vi "Actor.vi"(6 "Self Alias":string, 8 "Actor":refnum<class "Actor.lvclass">, 9 "Creator Attributes":T1, 10 "Queue of Created Init":refnum<queue>) -> ()   [LabVIEW 2020, in "jettl.lvlib" / "Actor.lvlib" / "Base Actor.lvclass"]
uses:
  Base Actor.lvclass
  Actor/Actor.lvclass
  Msg/Msg.lvclass
  Last Ack Msg/Last Ack Msg.lvlib
  Implemented Msgs.ctl
  Actor.lvlib
  Attributes.ctl
  Created Init.ctl
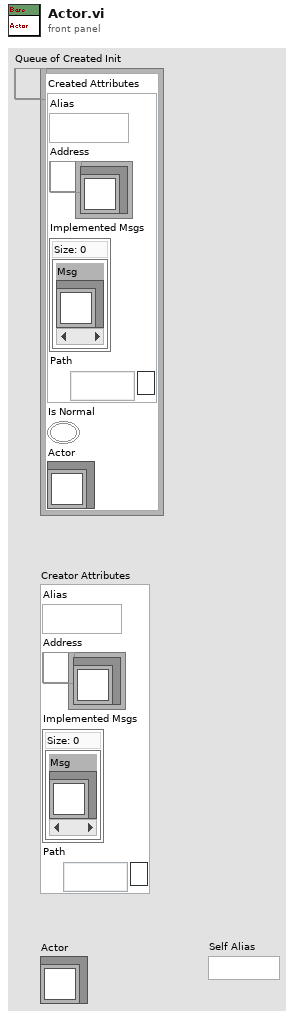
[diagram p1: front panel]
types:
  T1 = typedef "jettl.lvlib/Actor.lvlib/Attributes.ctl" = cluster{"Alias":string, "Address":refnum<user-event>, "Implemented Msgs":T2, "Path":path}
  T2 = typedef "jettl.lvlib/Actor.lvlib/Implemented Msgs.ctl" = set{refnum<class "Msg.lvclass">}
  T3 = typedef "jettl.lvlib/Actor.lvlib/Created Init.ctl" = cluster{"Created Attributes":T1, "Is Normal":bool, "Actor":refnum<class "Actor.lvclass">}
  T4 = typedef "jettl.lvlib/Actor.lvlib/Created Aliases.ctl" = set{string}
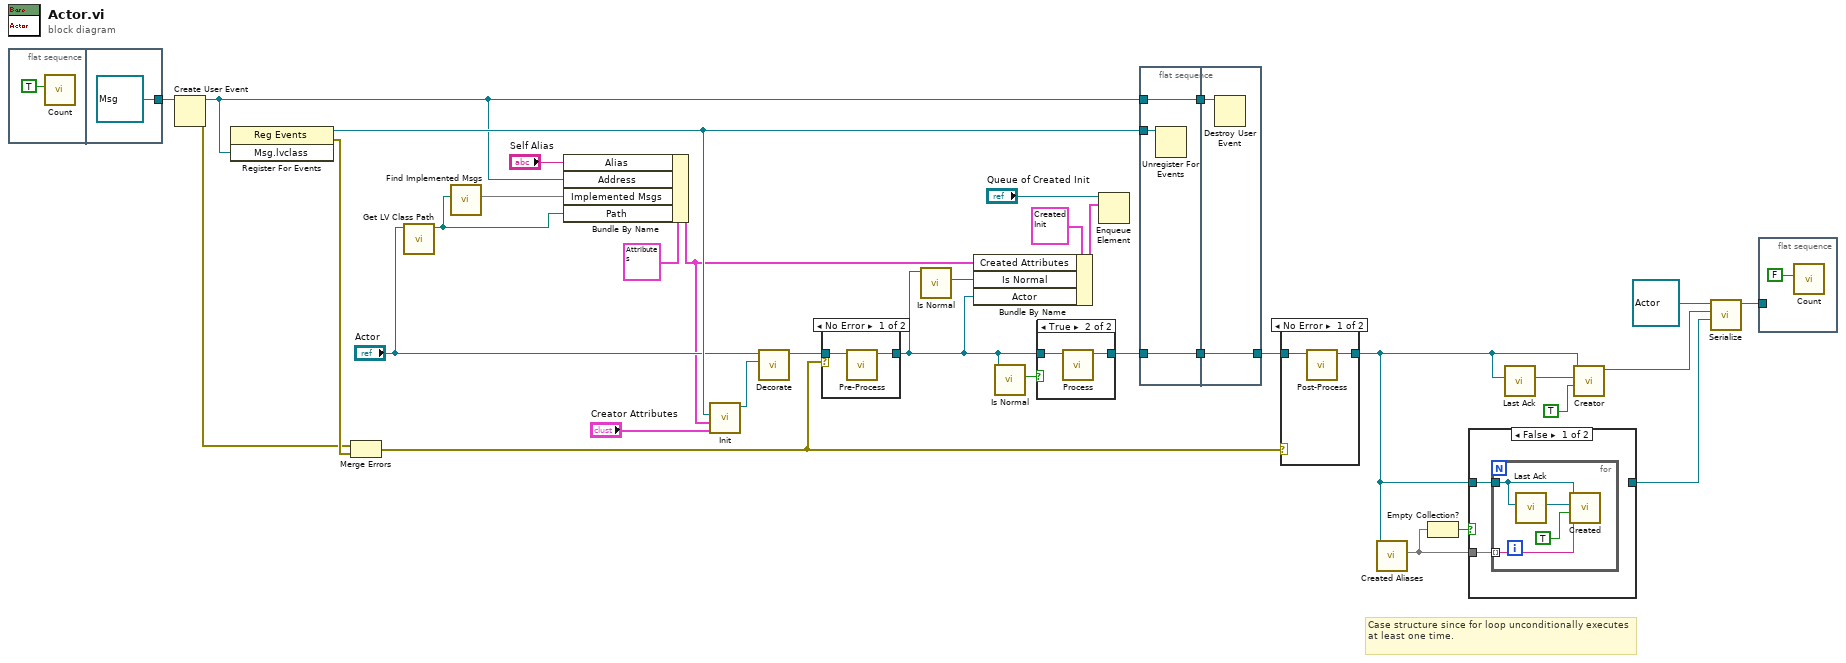
[diagram p0: block diagram]
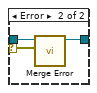
[diagram p5: hidden frame]
diagram:
  # "Case structure since for loop unconditionally executes at least one time."
  n1 = flat-sequence {
    tunnel: [refnum<class "Msg.lvclass"> refnum ("Msg.lvclass")] -> w32
    frame #0 {
      n2 = call "Count.vi"("Increment?"=TRUE) -> ()  [unwired: 11 in]
    }
    frame #1 {
    }
  }
  n3 = Create User Event(user event datatype=w32) -> (user event=w7:refnum<user-event>, error out=w33:errorcluster)  [unwired: 1 in]
  n4 = register-events(w7) -> (reference out=w14:refnum<event-registration>, error out=w34:errorcluster)  [unwired: 2 in]
  n5 = Merge Errors(w33, w34) -> (w25:errorcluster)
  n6 = call <vilib>:"Get LV Class Path.vi"("object"="Actor") -> ("class path"=w8:path)  [unwired: 9 in, 1 out]
  n7 = call "Find Implemented Msgs.vi"("Path"=w8) -> ("Implemented Msgs"=w9:T2)  [unwired: 10 in]
  n8 = Bundle By Name(cluster=T1 {"Alias"="", "Address"=refnum, "Implemented Msgs"={}, "Path"=path ""} ("Attributes"), "Alias"="Self Alias", "Address"=w7, "Implemented Msgs"=w9, "Path"=w8) -> (w1:T1)
  n9 = call "Init.vi"("Creator Attributes"="Creator Attributes", "Self Attributes"=w1, "Register"=w14) -> ("Base Actor out"=w31:refnum<class "Base Actor.lvclass">)  [unwired: 8 in]
  n10 = call-dynamic "Decorate.vi"("Actor"=w31, "Actor in"="Actor") -> ("Actor out"=w30:refnum<class "Actor.lvclass">)  [unwired: 9 in]
  n11 = case shown="No Error" w25 {
    selector: w25 -> [_ w39]
    tunnel: [w38 w40] -> w3
    tunnel: w30 -> [w37 w41]
    frame No Error {
      n12 = call-dynamic "Pre-Process.vi"("Actor in"=w37) -> ("Actor out"=w38:refnum<class "Actor.lvclass">)  [unwired: 10 in]
    }
    frame Error {
      n13 = call-dynamic "Merge Error.vi"("Error"=w39, "Actor in"=w41) -> ("Actor out"=w40:refnum<class "Actor.lvclass">)  [unwired: 9 in]
    }
  }
  n14 = call-dynamic "Is Normal.vi"("Actor in"=w3) -> ("Is Normal"=w2:bool)  [unwired: 10 in]
  n15 = Bundle By Name(cluster=T3 {"Created Attributes"={"Alias"="", "Address"=refnum, "Implemented Msgs"={}, "Path"=path ""}, "Is Normal"=FALSE, "Actor"=refnum} ("element"), "Created Attributes"=w1, "Is Normal"=w2, "Actor"=w3) -> (w4:T3)
  n16 = call-dynamic "Is Normal.vi"("Actor in"=w3) -> ("Is Normal"=w15:bool)  [unwired: 10 in]
  n17 = case shown="True" w15 {
    tunnel: w3 -> [w42 w44]
    tunnel: [w42 w43] -> w27
    frame False {
    }
    frame True {
      n18 = call-dynamic "Process.vi"("Actor in"=w44) -> ("Actor out"=w43:refnum<class "Actor.lvclass">)  [unwired: 10 in]
    }
  }
  n19 = Enqueue Element(queue="Queue of Created Init", element=w4) -> ()  [unwired: 2 in, 3 out]
  n20 = flat-sequence {
    tunnel: [w47] -> w28
    tunnel: w27 -> [w47]
    tunnel: w14 -> [w46]
    tunnel: w7 -> [w45]
    tunnel: [w45] -> w26
    tunnel: [w49] -> w29
    tunnel: w28 -> [w49]
    tunnel: w26 -> [w48]
    frame #0 {
      n21 = Unregister For Events(event registration refnum=w46) -> ()  [unwired: 1 in, 1 out]
    }
    frame #1 {
      n22 = Destroy User Event(user event=w48) -> ()  [unwired: 1 in, 1 out]
    }
  }
  n23 = case shown="No Error" w25 {
    tunnel: w29 -> [w51 w52]
    tunnel: [w50 w52] -> w19
    frame No Error {
      n24 = call-dynamic "Post-Process.vi"("Actor in"=w51) -> ("Actor out"=w50:refnum<class "Actor.lvclass">)  [unwired: 10 in]
    }
    frame Error {
    }
  }
  n25 = call-dynamic "Created Aliases.vi"("Actor in"=w19) -> ("Created Aliases"=w21:T4)  [unwired: 10 in]
  n26 = Empty Collection?(1:w21) -> (0:w22:bool)
  n27 = case shown="False" w22 {
    tunnel: w21 -> [w54 _]
    tunnel: w19 -> [w53 w59]
    tunnel: [_ w59] -> w17
    frame False {
      n28 = for {
        tunnel: w53 -> [w56]
        tunnel: w54 -> [w58] mode=indexing
        n29 = call "Last Ack.vi"("Actor"=w56) -> ("Msg"=w55:refnum<class "Msg.lvclass">)  [unwired: 10 in]
        n30 = call-dynamic "Created.vi"("Created Alias"=w58, "Is Priority"=TRUE ("Priority?"), "Msg"=w55, "Actor in"=w56) -> ()  [unwired: 7 in, 1 out]
      }
    }
    frame True {
    }
  }
  n31 = call "Last Ack.vi"("Actor"=w19) -> ("Msg"=w23:refnum<class "Msg.lvclass">)  [unwired: 10 in]
  n32 = call-dynamic "Creator.vi"("Is Priority"=TRUE ("Priority?"), "Msg"=w23, "Actor in"=w19) -> ("Actor out"=w18:refnum<class "Actor.lvclass">)  [unwired: 8 in]
  n33 = call-dynamic "Serialize.vi"("Input 2"=w17, "Input 1"=w18, "Actor in"=refnum<class "Actor.lvclass"> refnum ("jettl in")) -> ("Actor out"=w20:refnum<class "Actor.lvclass">)  [unwired: 8 in]
  n34 = flat-sequence {
    tunnel: w20 -> [_]
    frame #0 {
      n35 = call "Count.vi"("Increment?"=FALSE) -> ()  [unwired: 11 in]
    }
  }
